vi "Destructor.vi"(8 "error in (no error)":errorcluster, 11 "Shadow in":refnum<class "Shadow.lvclass">) -> (0 "error out":errorcluster)   [LabVIEW 2021, in "UIShadow.lvlib" / "Shadow.lvclass"]
uses:
  Shadow.lvclass
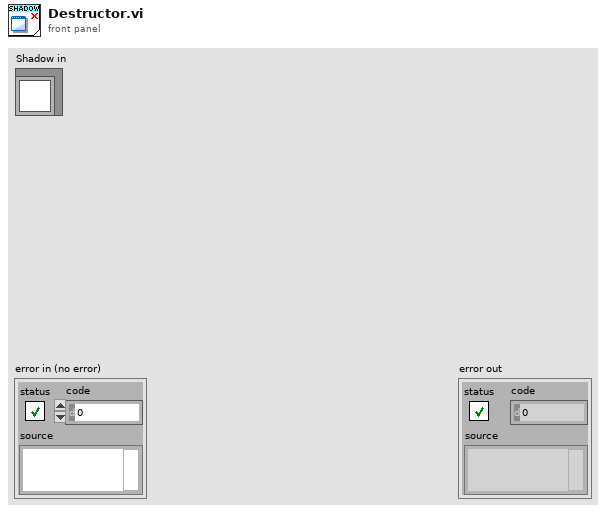
[diagram p1: front panel]
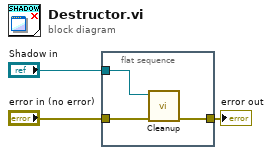
[diagram p0: block diagram]
diagram:
  n1 = flat-sequence {
    tunnel: "error in (no error)" -> [w6]
    tunnel: [w5] -> w2
    tunnel: "Shadow in" -> [w4]
    frame #0 {
      n2 = call "Cleanup.vi"("error in (no error)"=w6, "Shadow in"=w4) -> ("error out"=w5:errorcluster)  [unwired: 9 in]
    }
  }
  "error out" <- w2
